vi "get-action-type.vi"(11 "Subsytem name":string) -> ()   [LabVIEW 2017, in "automode.lvlib"]
uses:
  automode.lvlib
  <vilib>/regexp/Match Regular Expression.xnode
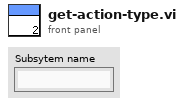
[diagram p1: front panel]
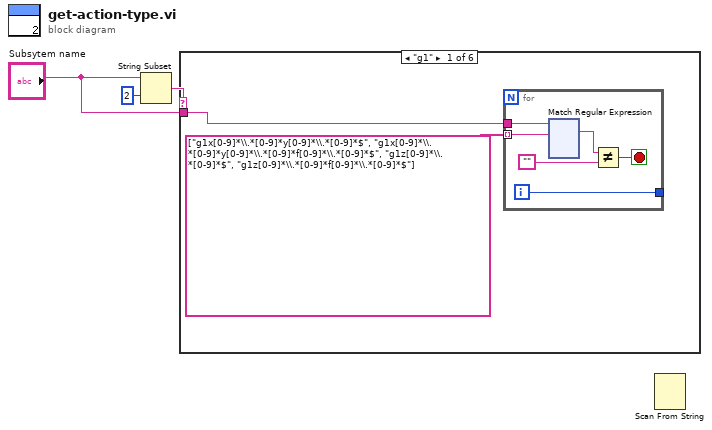
[diagram p0: block diagram]
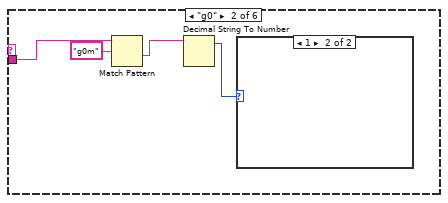
[diagram p2: hidden frame]
diagram:
  n1 = String Subset(string="Subsytem name", length (rest)=2 ("length (rest)")) -> (substring=w2:string)  [unwired: 1 in]
  n2 = case shown="\"g1\"" w2 {
    tunnel: "Subsytem name" -> [w4 w129 _ _ _ _]
    frame "g1" {
      n3 = for {
        tunnel: w4 -> [w9]
        tunnel: string[] ["g1x[0-9]*\\.*[0-9]*y[0-9]*\\.*[0-9]*$", "g1x[0-9]*\\.*[0-9]*y[0-9]*\\.*[0-9]*f[0-9]*\\.*[0-9]*$", "g1z[0-9]*\\.*[0-9]*$", "g1z[0-9]*\\.*[0-9]*f[0-9]*\\.*[0-9]*$"] -> [w8] mode=indexing
        tunnel: [w10] -> _
        i -> [w10]
        stop <- w11 stop-if-true
        n4 = xnode "Match Regular Expression"("input string"=w9, "regular expression"=w8) -> ("whole match"=w7:string)  [unwired: 4 in, 4 out]
        n5 = Not Equal?(x=w7, y="") -> (x != y?=w11:bool)
      }
    }
    frame "g0" {
      n6 = Match Pattern(string=w129, regular expression="g0m") -> (after substring=w127:string)  [unwired: 1 in, 3 out]
      n7 = Decimal String To Number(string=w127) -> (offset past number=w126:i32)  [unwired: 2 in, 1 out]
      n8 = case shown="1" w126 {
        frame 0, Default {
        }
        frame 1 {
        }
      }
    }
    frame "g2 " {
    }
    frame "g3" {
    }
    frame "t0" {
    }
    frame "t1" {
    }
  }
  n9 = Scan From String() -> ()  [unwired: 6 in, 3 out]
